vi "I2C_WriteBytesToSlave_2.vi"(5 "InterByteTransmitDelay(Ticks)":u32, 7 "HalfCycle(Ticks)":u32, 8 "error in":errorcluster, 10 "StatusIn":i16, 11 "NumBytesToWrite":i32) -> (0 "error out":errorcluster, 2 "Status":i16)   [LabVIEW 2019]
doc: "Writes Data bytes out the I2C Bus\n\n<b>Inputs:</b>\n---------------------\n<b>NumBytesToWrite</b> the number of bytes to read from the 'Write' memory block of the FPGA starting at index 0.\n\n<b>HalfCycle(Ticks)</b> this the number of FPGA clock cycles in half og the clock period. Therefore twice this number yields the clock period, in ticks.\n\n<b>TransmitDelay(Ticks)</b> the delay in FPGA clock cycles before writing bytes on SDA.\n\n<b>StatusIn</b> the status of the Slave Device / I2C Bus\n\n<b>Outputs:</b>\n---------------------\n<b>Status</b> returns a numeric value representing the status of the I2C bus / slave device.\n0 = slave responded\n5002 = slave did not respond\n\nSee block diagram for more details on the implementation details.\n\nAuthor:\nPeter Fuller\nSenior Engineer\nPLF Consulting, LLC\n\nemail: peter@plfconsulting.com\nphone: 617.699.2201"
uses:
  <vilib>/rvi/DataTransferAndStorage/Container/XNode/niFpgaContainer.xnode
  <vilib>/rvi/Memory/Memory_Emulation/nirvimemoryEmulation.vi
  <vilib>/rvi/Memory/Memory_Emulation/nirvimemoryFastEmulation.vi
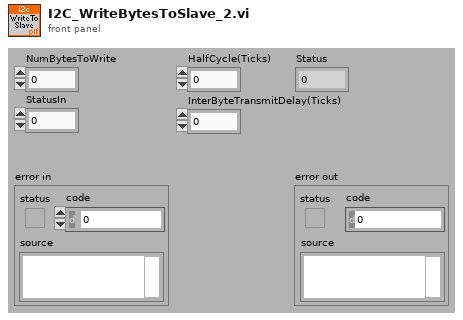
[diagram p1: front panel]
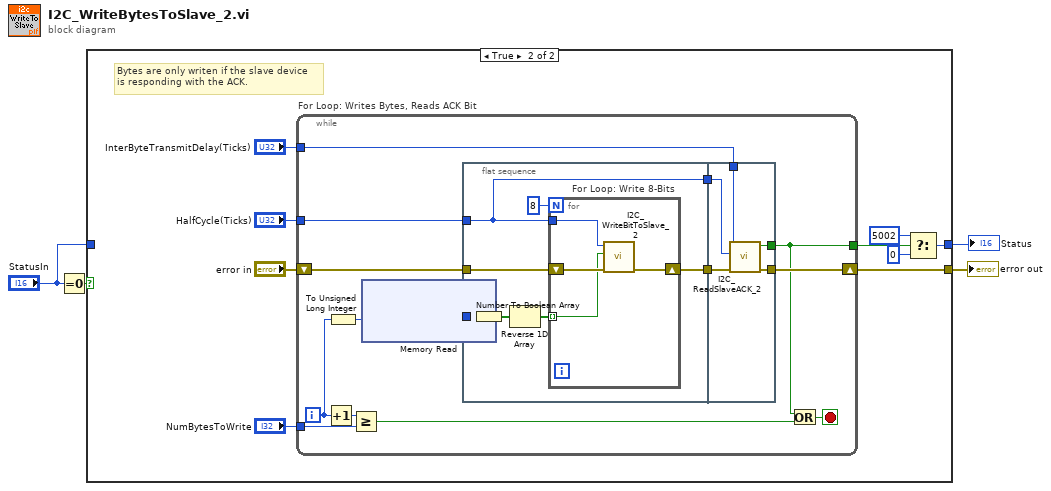
[diagram p0: block diagram]
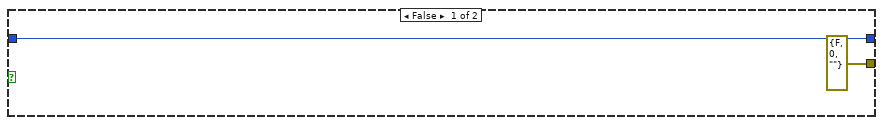
[diagram p2: hidden frame]
diagram:
  n1 = Equal To 0?(x="StatusIn") -> (x = 0?=w2:bool)
  n2 = case shown="True" w2 {
    tunnel: [errorcluster {"status"=FALSE, "code"=0, "source"=""} ("error in") w14] -> w4
    tunnel: [w6 w7] -> w3
    tunnel: "StatusIn" -> [w6 _]
    frame False {
    }
    frame True {
      # "Bytes are only writen if the slave device\nis responding with the ACK."
      n3 = while "For Loop: Writes Bytes, Reads ACK Bit" {
        tunnel: "HalfCycle(Ticks)" -> [w17]
        shift-right: [w19] -> w14
        shift-left: "error in" -> [w29]
        tunnel: "NumBytesToWrite" -> [w26]
        tunnel: [w16] -> w10
        tunnel: "InterByteTransmitDelay(Ticks)" -> [w20]
        i -> [w25]
        stop <- w28 stop-if-true
        n4 = Increment(x=w25) -> (x+1=w27:i32)
        n5 = To Unsigned Long Integer(number=w25) -> (unsigned 32bit integer=w24:u32)
        n6 = Greater Or Equal?(x=w27, y=w26) -> (x >= y?=w23:bool)
        n7 = xnode ("Memory Read")("Address"=w24) -> ("Data"=w21:u8)  [unwired: 1 in, 1 out]
        n8 = flat-sequence {
          tunnel: w17 -> [w30]
          tunnel: w29 -> [w33]
          tunnel: w21 -> [w31]
          tunnel: [w32] -> w22
          tunnel: [w30] -> w18
          tunnel: w22 -> [w44]
          tunnel: w20 -> [w45]
          tunnel: [w43] -> w19
          tunnel: [w42] -> w16
          tunnel: w18 -> [w41]
          frame #0 {
            n9 = Number To Boolean Array(number=w31) -> (Boolean array=w35:bool[])
            n10 = Reverse 1D Array(array=w35) -> (reversed array=w34:bool[])
            n11 = for "For Loop: Write 8-Bits" {
              N: 8 -> [_]
              tunnel: w34 -> [w38] mode=indexing
              shift-right: [w37] -> w32
              shift-left: w33 -> [w40]
              tunnel: w30 -> [w39]
              n12 = call "I2C_WriteBitToSlave_2.vi"("error in"=w40, "Bit_Value"=w38, "HalfCycle(Ticks)"=w39) -> ("error out"=w37:errorcluster)  [unwired: 8 in]
            }
          }
          frame #1 {
            n13 = call "I2C_ReadSlaveACK_2.vi"("error in"=w44, "HalfCycle(Ticks)"=w41, "InterByteTransmitDelay(Ticks)"=w45) -> ("error out"=w43:errorcluster, "SDA"=w42:bool)  [unwired: 7 in]
          }
        }
        n14 = Or(x=w16, y=w23) -> (x .or. y?=w28:bool)
      }
      n15 = Select(t=i16 5002, s=w10, f=i16 0) -> (s? t:f=w7:i16)
    }
  }
  "error out" <- w4
  "Status" <- w3
